vi "libssh2_agent_sign.vi"(8 "error in (no error)":errorcluster, 9 "data":u8[](array[numeric]), 10 "identity":T1, 11 "agent":T2) -> (0 "error out":errorcluster, 2 "signature":u8[](array[numeric]))   [LabVIEW 2013, in "libssh2.lvlib"]
doc: "Sign a buffer with a public key from an SSH agent."
uses:
  libssh2.lvlib
  Agent Refnum.ctl
  Agent Public Key Refnum.ctl
  Not An Agent.vi
  <vilib>/Utility/error.llb/Error Cluster From Error Code.vi
  Not An Agent Public Key.vi
  Global Settings.vi
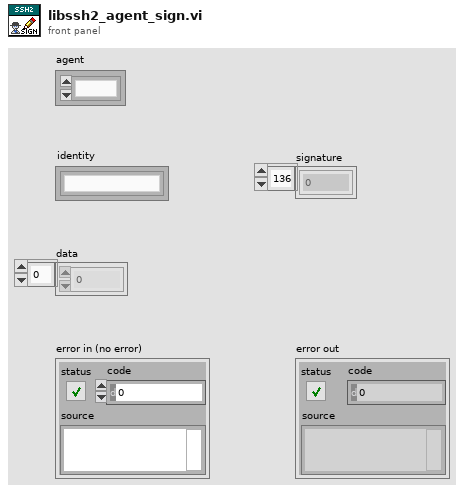
[diagram p1: front panel]
types:
  T1 = typedef "libssh2.lvlib/Agent Public Key Refnum.ctl" = refnum<k1>
  T2 = typedef "libssh2.lvlib/Agent Refnum.ctl" = refnum<k1>
  T3 = typedef "libssh2.lvlib/libssh2_agent_publickey.ctl" = cluster{"magic":i32, "node":u64, "blob":u8[], "blob_len":i32, "comment":string}
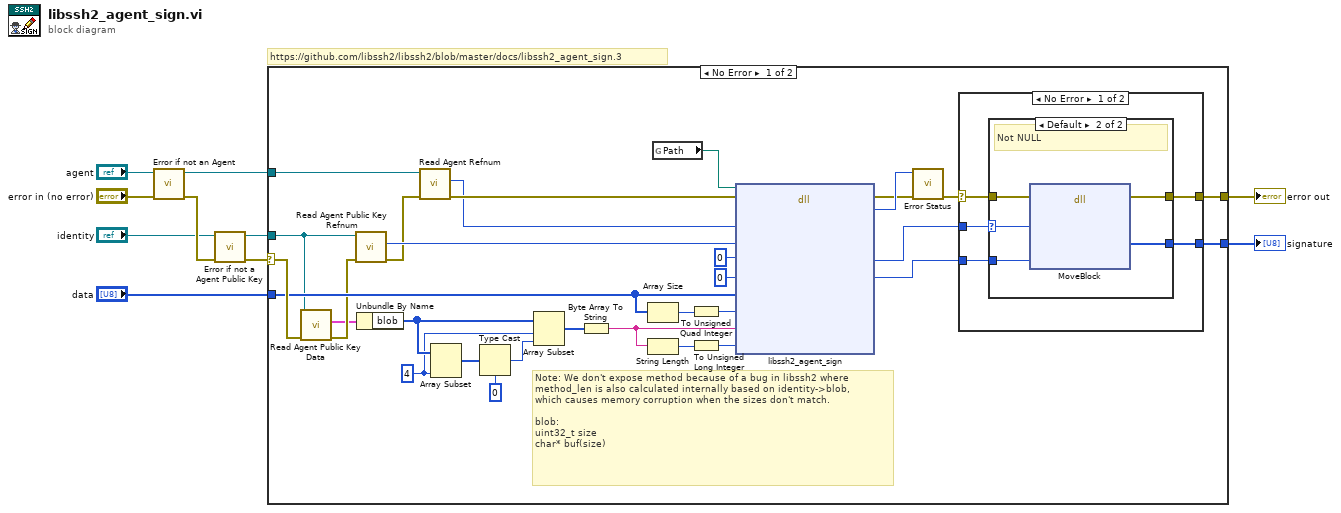
[diagram p0: block diagram]
diagram:
  # "https://github.com/libssh2/libssh2/blob/master/docs/libssh2_agent_sign.3"
  n1 = call "Error if not an Agent.vi"("error in (no error)"="error in (no error)", "agent"="agent") -> ("error out"=w6:errorcluster, "agent out"=w7:T2)  [unwired: 8 in]
  n2 = call "Error if not a Agent Public Key.vi"("error in (no error)"=w6, "agent public key"="identity") -> ("error out"=w5:errorcluster, "agent public key out"=w3:T1)  [unwired: 8 in]
  n3 = case shown="No Error" w5 {
    selector: w5 -> [w35 w53]
    tunnel: [w23 w53] -> w10
    tunnel: w7 -> [w41 _]
    tunnel: w3 -> [w19 _]
    tunnel: "data" -> [w32 _]
    tunnel: [w22 _] -> w1
    frame No Error {
      w13 = 4 ("length")
      # "Note: We don't expose method because of a bug in libssh2 where method_len is also calculated internally based on identity->blob,\nwhich causes memory corruption when the sizes don't match.\n\nblob:\nuint32_t size\nchar* buf(size)"
      n4 = call "Read Agent Public Key Data.vi"("error in (no error)"=w35, "agent public key"=w19) -> ("error out"=w20:errorcluster, "value"=w18:T3)  [unwired: 8 in]
      n5 = call "Read Agent Public Key Refnum.vi"("error in (no error)"=w20, "agent public key"=w19) -> ("error out"=w34:errorcluster, "libssh2_agent_publickey*"=w36:u64)  [unwired: 8 in]
      n6 = Unbundle By Name(w18) -> ("blob"=w15:u8[])
      n7 = call "Read Agent Refnum.vi"("error in (no error)"=w34, "agent"=w41) -> ("error out"=w38:errorcluster, "LIBSSH2_AGENT*"=w37:u64)  [unwired: 8 in]
      n8 = Array Subset(array=w15, length=w13) -> (w17:u8[])  [unwired: 1 in]
      n9 = Type Cast(type=u32 0, x=w17) -> (*(type *) &x=w14:u32)
      n10 = Array Subset(array=w15, index=w13, length=w14) -> (w12:u8[])
      n11 = Byte Array To String(unsigned byte array=w12) -> (string=w11:string)
      n12 = Array Size(array=w32) -> (size(s)=w31:i32)
      n13 = String Length(string=w11) -> (length=w29:i32)
      n14 = global read "Global Settings.vi" "Path"() -> (w39:path)
      n15 = To Unsigned Quad Integer(1:w31) -> (0:w30:u64)
      n16 = To Unsigned Long Integer(number=w29) -> (unsigned 32bit integer=w28:u32)
      n17 = dll-call lib="?" fn="libssh2_agent_sign"(path in=w39, error in=w38, "agent"=w37, "identity"=w36, "sig"=u64 0, "s_len"=u64 0, "data"=w32, "d_len"=w30, "method"=w11, "method_len"=w28) -> (error out=w27:errorcluster, "return value"=w40:i32, "sig"=w25:u64, "s_len"=w24:u64)  [unwired: 7 in, 1 out]
      n18 = call "Error Status.vi"("error in (no error)"=w27, "return value"=w40) -> ("error out"=w21:errorcluster)  [unwired: 8 in, 1 out]
      n19 = case shown="No Error" w21 {
        selector: w21 -> [w42 w52]
        tunnel: w25 -> [w46 _]
        tunnel: w24 -> [w45 _]
        tunnel: [w44 w52] -> w23
        tunnel: [w43 _] -> w22
        frame No Error {
          n20 = case shown="Default" w46 {
            selector: w46 -> [_ w48]
            tunnel: w45 -> [_ w51]
            tunnel: [_ w50] -> w43
            tunnel: [_ w49] -> w44
            tunnel: w42 -> [_ w47]
            frame 0 {
              # "NULL"
            }
            frame Default {
              # "Not NULL"
              n21 = dll-call lib="LabVIEW" fn="MoveBlock"(error in=w47, "ps"=w48, "size"=w51) -> (error out=w49:errorcluster, "pd"=w50:u8[])  [unwired: 6 in, 1 out]
            }
          }
        }
        frame Error {
        }
      }
    }
    frame Error {
    }
  }
  "error out" <- w10
  "signature" <- w1
